vi "写入消息.vi"(8 "error in (no error)":errorcluster caption="错误输入（无错误）", 10 "消息":string, 11 "消息类输入":refnum<class "消息类.lvclass">) -> (0 "error out":errorcluster caption="错误输出", 3 "消息类输出":refnum<class "消息类.lvclass">)   [LabVIEW 2016, in "消息类.lvclass"]
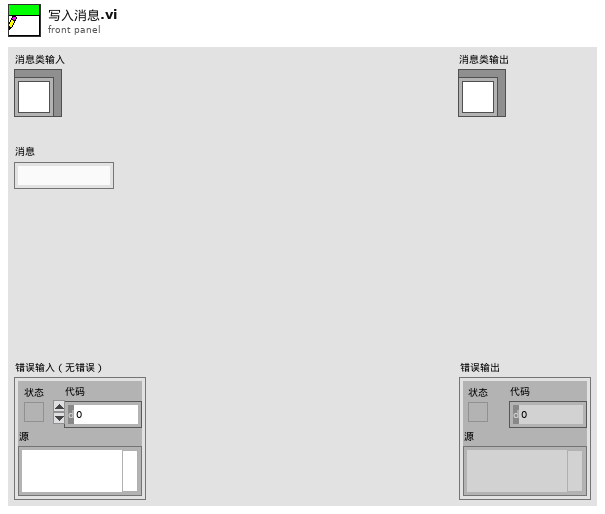
[diagram p1: front panel]
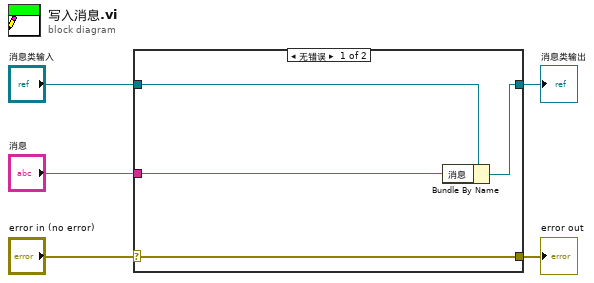
[diagram p0: block diagram]
diagram:
  n1 = case shown="无错误" "error in (no error)" {
    selector: "error in (no error)" -> [w9 w10]
    tunnel: [w9 w10] -> w4
    tunnel: [w7 w11] -> w2
    tunnel: "消息类输入" -> [w8 w11]
    tunnel: "消息" -> [w6 _]
    frame No Error {
      n2 = Bundle By Name(cluster=w8, "消息"=w6) -> (w7:refnum<class "消息类.lvclass">)
    }
    frame Error {
    }
  }
  "error out" <- w4
  "消息类输出" <- w2
